vi "GUI MAIN.vi"() -> ()   [LabVIEW 2022 SP3]
uses:
  <vilib>/Instr/_visa.llb/VISA Configure Serial Port (Instr).vi
panel:
  out "Selected Freq":i32
  in  "Send":bool
  out "Send return count":u32
  in  "stop":bool
  in  "input cluster":T1
  out "read buffer":string
  out "return count":u32
  in  "VISA resource name":refnum<visa-resource-name>
  in  "FT DataSize":i32
  out "Fourier Transform":cluster{i32, dbl, i32[][]}(graph)
  out "Intensity Chart":i32[][](graph)
  out "Thermometer 5":i32(slide) scale=20.0..20000.0
  in  "Signal 5":bool
  out "Thermometer 4":i32(slide) scale=20.0..20000.0
  out "Thermometer 3":i32(slide) scale=20.0..20000.0
  out "Thermometer 2":i32(slide) scale=20.0..20000.0
  out "Thermometer 1":i32(slide) scale=20.0..20000.0
  in  "Signal 4":bool
  in  "Signal 3":bool
  in  "Signal 2":bool
  in  "Signal 1":bool
  out "Radar Graph":i32[][](graph)
  # "Signature Selection"
  # "Frequency (Hz)"
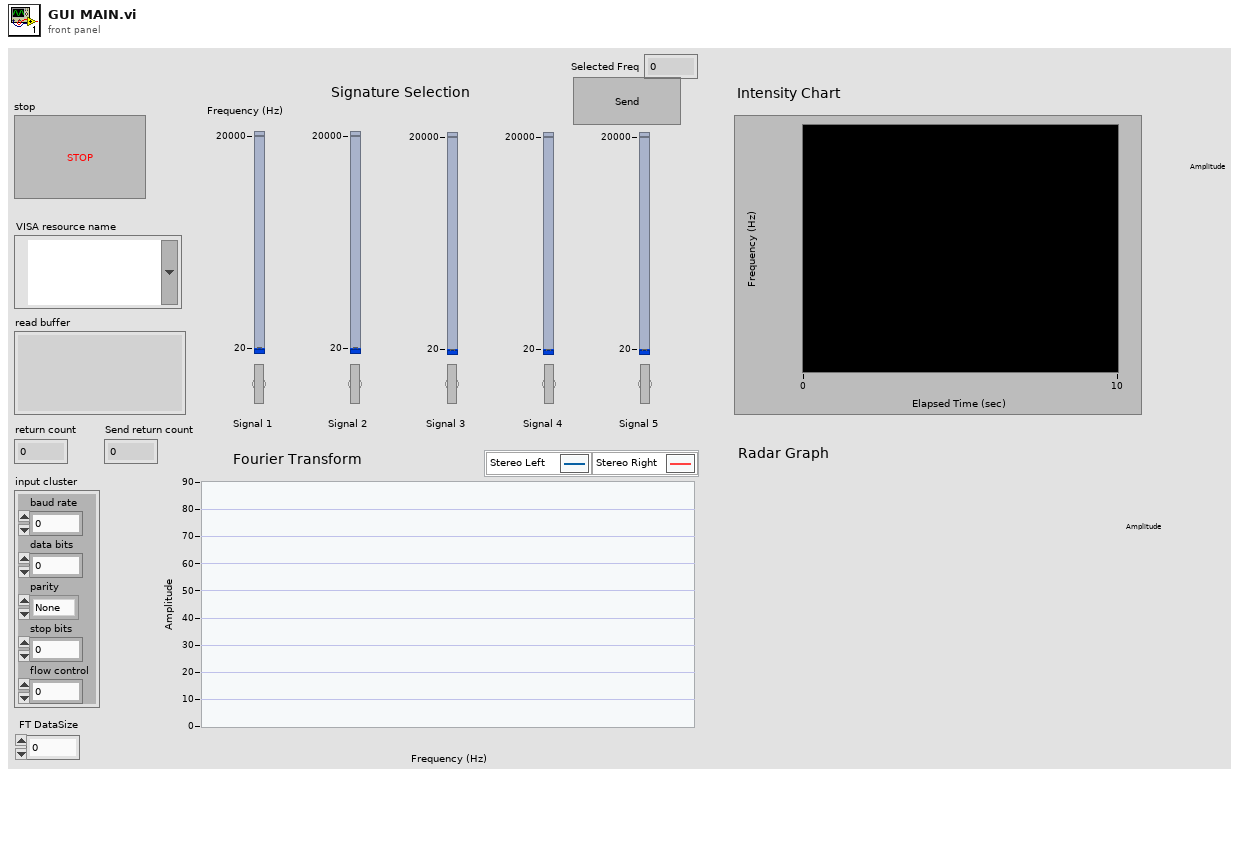
[diagram p1: front panel]
types:
  T1 = cluster{"baud rate":u32, "data bits":u16, "parity":enum16{"None", "Odd", "Even", "Mark", "Space"}, "stop bits":u16, "flow control":u16}
  T2 = cluster{"Width":u16, "Style":enum32{"Solid", "Dash", "Dot", "DashDot", "DashDotDot"}}
  T3 = typedef "LVRectTypeDef.ctl" = cluster{"left":i16, "top":i16, "right":i16, "bottom":i16}
  T4 = typedef "LVPoint32TypeDef.ctl" = cluster{"Horizontal":i32, "Vertical":i32}
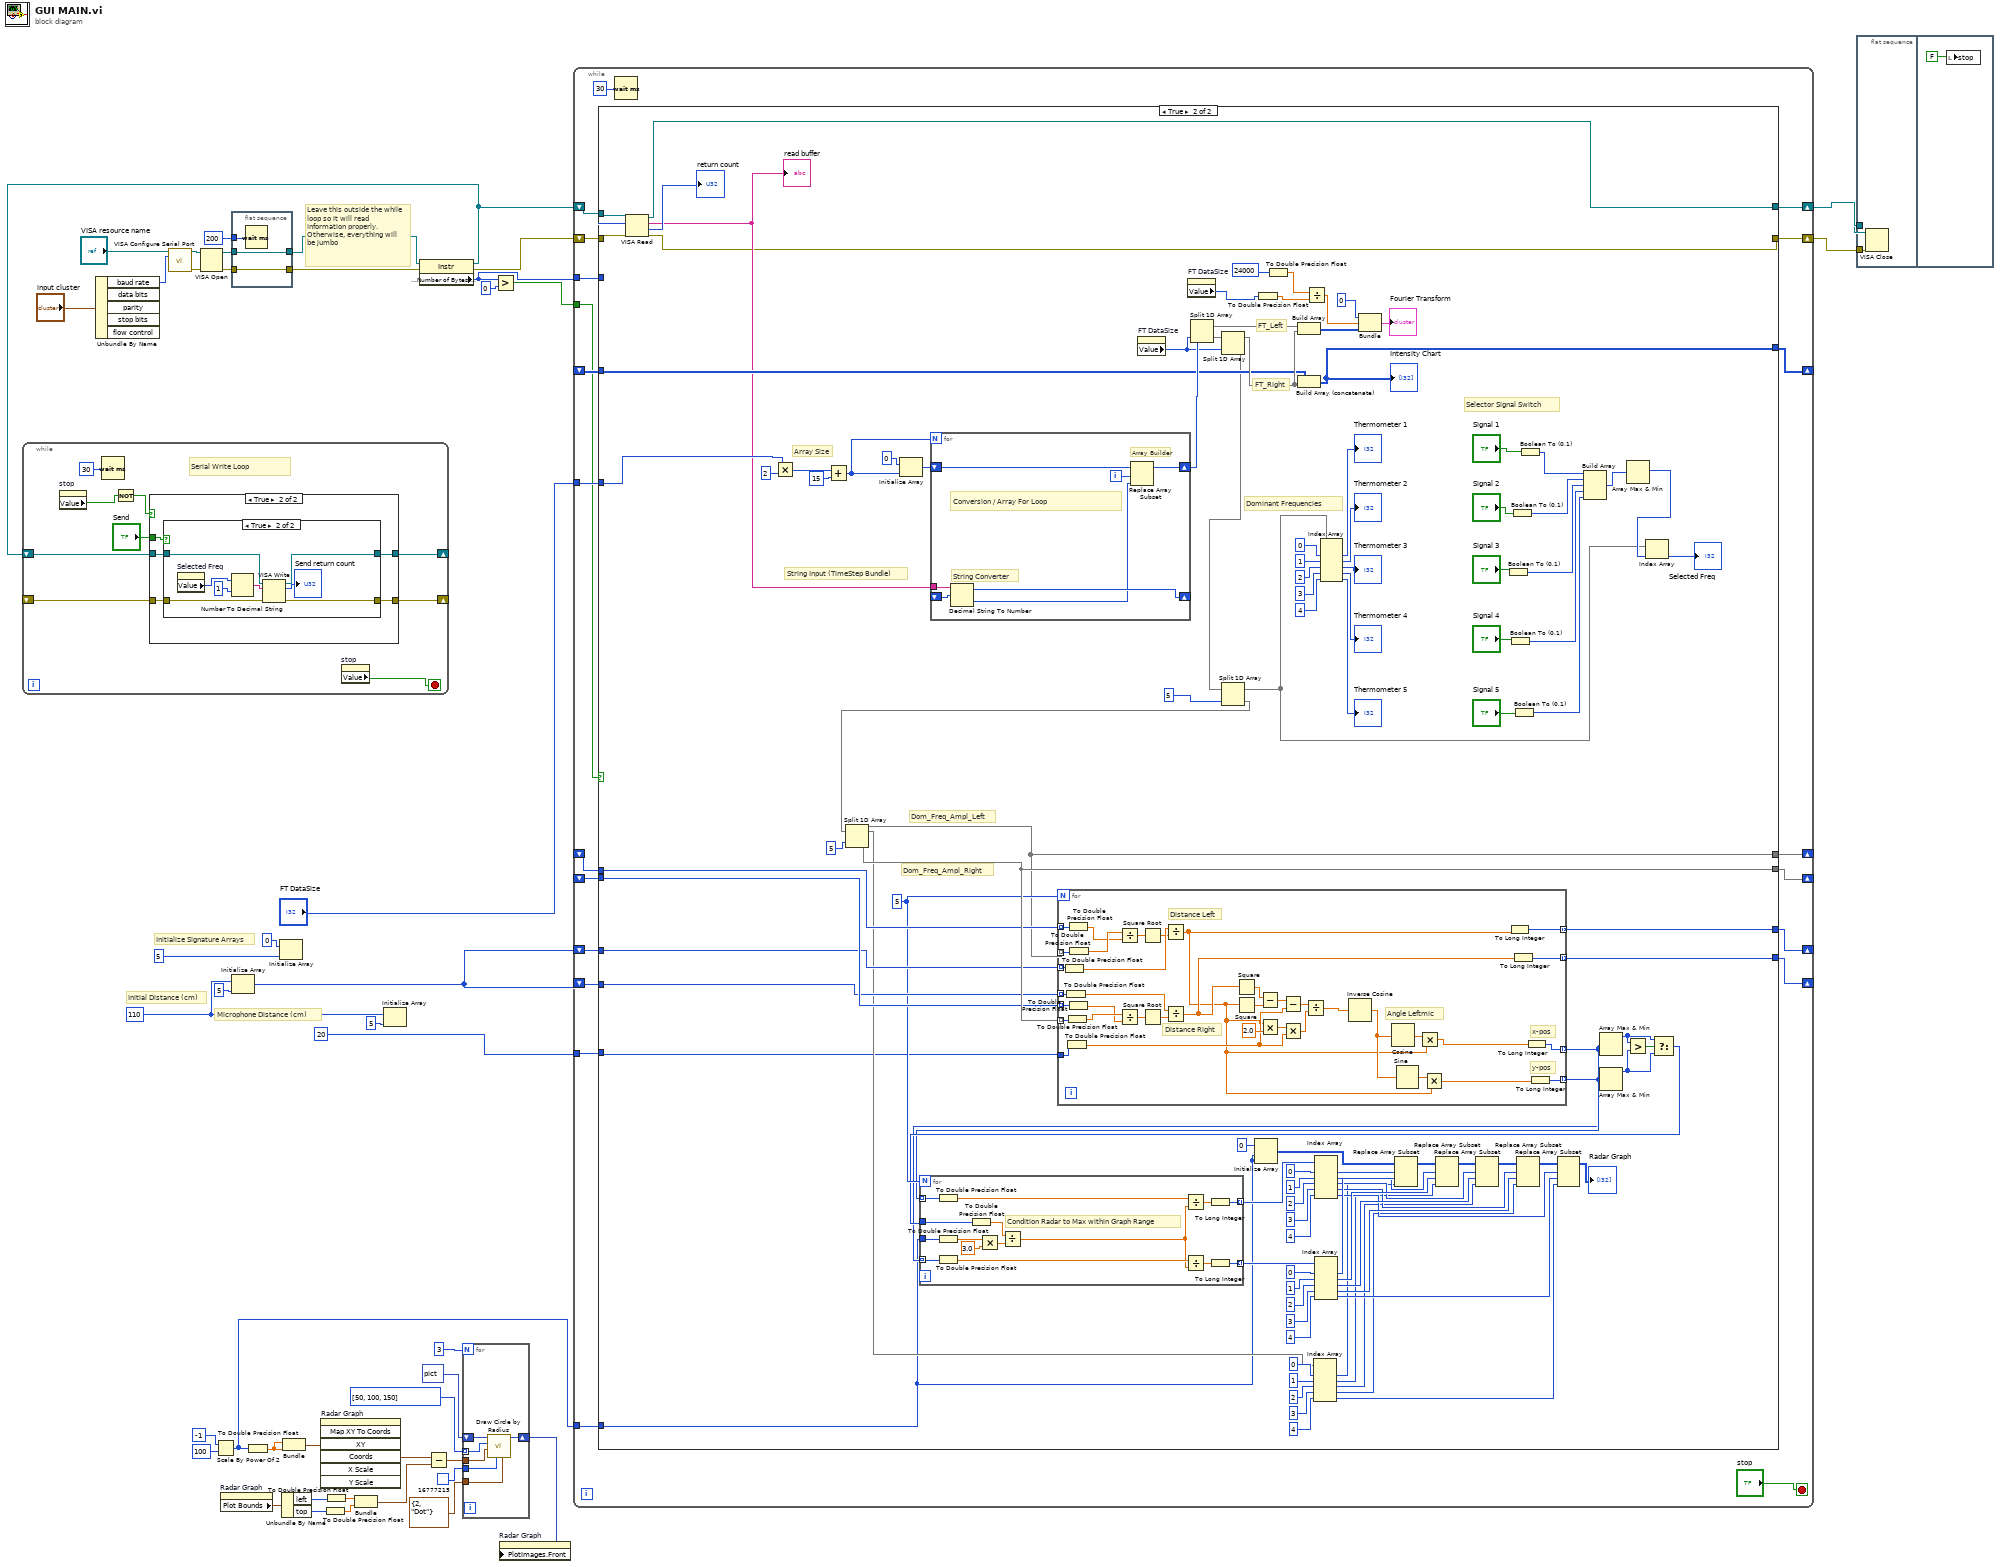
[diagram p0: block diagram]
diagram:
  w27 = 110
  # "Leave this outside the while loop so it will read information properly. Otherwise, everything will be jumbo"
  # "Initialize Signature Arrays"
  # "Microphone Distance (cm)"
  # "Initial Distance (cm)"
  n1 = Unbundle By Name("input cluster") -> ("baud rate"=w19:u32)  [unwired: 4 out]
  n2 = call-poly "VISA Configure Serial Port"("VISA resource name"="VISA resource name", "baud rate (9600)"=w19) -> ("VISA resource name out"=w17:refnum<visa-resource-name>, "error out"=w16:errorcluster)  [unwired: 12 in]
  n3 = VISA Open(error in (no error)=w16, VISA resource name=w17) -> (VISA resource name=w24:refnum<visa-resource-name>, error out=w23:errorcluster)  [unwired: 3 in]
  n4 = Scale By Power Of 2(n=-1, x=100 ("samples")) -> (x*2^n=w1:i32)
  n5 = property on="Radar Graph" class="IntGraph (strict)"() -> ("Plot Bounds"=w35:T3)  [unwired: 2 in, 2 out]
  n6 = flat-sequence {
    tunnel: w23 -> [w46]
    tunnel: [w46] -> w15
    tunnel: w24 -> [w45]
    tunnel: [w45] -> w20
    tunnel: u32 200 -> [w47]
    frame #0 {
      n7 = Wait (ms)(milliseconds to wait=w47) -> ()  [unwired: 1 out]
    }
  }
  n8 = Initialize Array(w27, 5) -> (w30:i32[])
  n9 = To Double Precision Float(number=w1) -> (double precision float=w8:dbl)
  n10 = Initialize Array(0, 5) -> ()  [unwired: 1 out]
  n11 = Unbundle By Name(w35) -> ("left"=w6:i16, "top"=w4:i16)
  n12 = Bundle(w8, w8) -> (w7:cluster{dbl, dbl})  [unwired: 1 in]
  n13 = invoke on="Radar Graph" class="IntGraph (strict)" method="Map XY To Coords"("XY"=w7) -> ("Coords"=w2:T4)  [unwired: 6 in, 6 out]
  n14 = To Double Precision Float(number=w4) -> (double precision float=w3:dbl)
  n15 = To Double Precision Float(number=w6) -> (double precision float=w5:dbl)
  n16 = Bundle(w5, w3) -> (w34:cluster{dbl, dbl})  [unwired: 1 in]
  n17 = Initialize Array(w27, 5) -> ()  [unwired: 1 out]
  n18 = property class="Instr"(reference=w20, error in=w15) -> (reference out=w9:refnum<visa-resource-name>, error out=w11:errorcluster, "Serial Settings:Number of Bytes at Serial Port"=w12:u32)
  n19 = while {
    shift-right: [w55] -> _
    shift-left: w9 -> [w56]
    shift-right: [w52] -> _
    shift-left: _ -> [w53]
    stop <- w48 stop-if-true
    # "Serial Write Loop"
    n20 = property on="stop" class="Bool (strict)"() -> ("Value"=w51:bool)  [unwired: 2 in, 2 out]
    n21 = Wait (ms)(milliseconds to wait=u32 30) -> ()  [unwired: 1 out]
    n22 = Not(x=w51) -> (.not. x?=w50:bool)
    n23 = case shown="True" w50 {
      tunnel: w56 -> [w58 w62]
      tunnel: [w58 w59] -> w55
      tunnel: w53 -> [w57 w61]
      tunnel: [w57 w60] -> w52
      tunnel: "Send" -> [_ w63]
      frame False {
      }
      frame True {
        n24 = case shown="True" w63 {
          tunnel: w62 -> [w65 w70]
          tunnel: w61 -> [w64 w69]
          tunnel: [w64 w67] -> w60
          tunnel: [w65 w68] -> w59
          frame False {
          }
          frame True {
            n25 = property on="Selected Freq" class="DigNum (strict)"() -> ("Value"=w66:i32)  [unwired: 2 in, 2 out]
            n26 = Number To Decimal String(number=w66, width (-)=i16 1) -> (decimal integer string=w72:string)
            n27 = VISA Write(VISA resource name=w70, write buffer=w72, error in (no error)=w69) -> (VISA resource name out=w68:refnum<visa-resource-name>, return count=→"Send return count":u32, error out=w67:errorcluster)
          }
        }
      }
    }
    n28 = property on="stop" class="Bool (strict)"() -> ("Value"=w48:bool)  [unwired: 2 in, 2 out]
  }
  n29 = Subtract(x=w2, y=w34) -> (x-y=w36:cluster{dbl, dbl})
  n30 = for {
    N: 3 -> [_]
    tunnel: w36 -> [w79]
    tunnel: u32 16777215 ("color(black)") -> [w78]
    tunnel: T2 {"Width"=2, "Style"=enum."Dot"} ("pen") -> [w77]
    tunnel: i16[] [50, 100, 150] -> [w76] mode=indexing
    shift-right: [w74] -> w38
    shift-left: picture data[5B] ("new picture") -> [w75]
    n31 = call <vilib>:"Draw Circle by Radius.vi"("pen"=w77, "color(black)"=w78, "pixel center"=w79, "radius"=w76, "picture"=w75) -> ("new picture"=w74:picture)  [unwired: 6 in]
  }
  n32 = Greater?(x=w12, y=u32 0) -> (0:w10:bool)
  n33 = property on="Radar Graph" class="IntGraph (strict)"("PlotImages.Front"=w38) -> ()  [unwired: 2 in, 2 out]
  n34 = while {
    shift-right: [w80] -> _
    shift-left: _ -> [w100]
    tunnel: "FT DataSize" -> [w99]
    tunnel: 20 -> [w83]
    shift-right: [w87] -> _
    shift-left: _ -> [w91]
    shift-right: [w86] -> _
    shift-left: _ -> [w92]
    shift-right: [w85] -> _
    shift-left: w30 -> [w90]
    shift-right: [w84] -> _
    shift-left: w30 -> [w89]
    shift-right: [w82] -> w14
    shift-left: w9 -> [w96]
    shift-right: [w81] -> w13
    shift-left: w11 -> [w95]
    tunnel: w12 -> [w94]
    tunnel: w10 -> [w93]
    tunnel: w1 -> [w88]
    stop <- "stop" stop-if-true
    n35 = case shown="True" w93 {
      tunnel: w100 -> [w105 w211]
      tunnel: [w105 w210] -> w80
      tunnel: w99 -> [_ w195]
      tunnel: [w103 w189] -> w86
      tunnel: w91 -> [w104 w188]
      tunnel: w92 -> [w103 w187]
      tunnel: w90 -> [w102 w186]
      tunnel: w89 -> [w101 w185]
      tunnel: [w101 w184] -> w84
      tunnel: [w102 w183] -> w85
      tunnel: w83 -> [_ w126]
      tunnel: [w104 w143] -> w87
      tunnel: w96 -> [w107 w131]
      tunnel: w95 -> [w106 w130]
      tunnel: w94 -> [_ w128]
      tunnel: w88 -> [_ w124]
      tunnel: [w107 w114] -> w82
      tunnel: [w106 w113] -> w81
      frame False {
      }
      frame True {
        w182 = 5
        # "String Input (TimeStep Bundle)"
        # "Selector Signal Switch"
        # "Dom_Freq_Ampl_Right"
        # "Dom_Freq_Ampl_Left"
        # "Dominant Frequencies"
        # "FT_Right"
        # "FT_Left"
        # "Array Size"
        n36 = VISA Read(VISA resource name=w131, byte count=w128, error in (no error)=w130) -> (VISA resource name out=w114:refnum<visa-resource-name>, read buffer=w125:string, return count=→"return count":u32, error out=w113:errorcluster)
        "read buffer" <- w125
        n37 = Multiply(x=w195, y=2) -> (x*y=w193:i32)
        n38 = Add(x=w193, y=15) -> (x+y=w191:i32)
        n39 = Initialize Array(0, w191) -> (w219:i32[])
        n40 = for {
          N: w191 -> [_]
          tunnel: w125 -> [w279]
          shift-right: [w278] -> _
          shift-left: _ -> [w277]
          shift-right: [w276] -> w218
          shift-left: w219 -> [w275]
          i -> [w273]
          # "String Converter"
          # "Array Builder"
          # "Conversion / Array For Loop"
          n41 = Decimal String To Number(string=w279, offset=w277) -> (offset past number=w278:i32, number=w274:i32)  [unwired: 1 in]
          n42 = Replace Array Subset(array=w275, new element=w274, index=w273) -> (w276:i32[])
        }
        n43 = property on="FT DataSize" class="DigNum (strict)"() -> ("Value"=w190:i32)  [unwired: 2 in, 2 out]
        n44 = property on="FT DataSize" class="DigNum (strict)"() -> ("Value"=w109:i32)  [unwired: 2 in, 2 out]
        n45 = Split 1D Array(array=w218, index=w190) -> (first subarray=w216:i32[], second subarray=w217:i32[])
        n46 = Split 1D Array(array=w217, index=w190) -> (first subarray=w212:i32[], second subarray=w199:i32[])
        n47 = Split 1D Array(array=w199, index=5) -> (first subarray=w116:i32[], second subarray=w196:i32[])
        n48 = Split 1D Array(array=w196, index=5) -> (first subarray=w143:i32[], second subarray=w189:i32[])
        n49 = for {
          N: w182 -> [_]
          tunnel: w143 -> [w270] mode=indexing
          tunnel: w189 -> [w269] mode=indexing
          tunnel: w188 -> [w272] mode=indexing
          tunnel: w187 -> [w271] mode=indexing
          tunnel: w186 -> [w262] mode=indexing
          tunnel: w185 -> [w261] mode=indexing
          tunnel: [w255] -> w184 mode=indexing
          tunnel: [w256] -> w183 mode=indexing
          tunnel: w126 -> [w254]
          tunnel: [w237] -> w177 mode=indexing
          tunnel: [w238] -> w176 mode=indexing
          # "y-pos"
          # "x-pos"
          # "Angle Leftmic"
          # "Distance Right"
          # "Distance Left"
          n50 = To Double Precision Float(number=w262) -> (double precision float=w260:dbl)
          n51 = To Double Precision Float(number=w261) -> (double precision float=w258:dbl)
          n52 = To Double Precision Float(number=w254) -> (double precision float=w247:dbl)
          n53 = To Double Precision Float(number=w269) -> (double precision float=w266:dbl)
          n54 = To Double Precision Float(number=w272) -> (double precision float=w267:dbl)
          n55 = To Double Precision Float(number=w271) -> (double precision float=w265:dbl)
          n56 = To Double Precision Float(number=w270) -> (double precision float=w268:dbl)
          n57 = Divide(x=w268, y=w267) -> (x/y=w263:dbl)
          n58 = Divide(x=w266, y=w265) -> (x/y=w264:dbl)
          n59 = Square Root(x=w263) -> (sqrt(x)=w259:dbl)
          n60 = Square Root(x=w264) -> (sqrt(x)=w257:dbl)
          n61 = Divide(x=w260, y=w259) -> (x/y=w240:dbl)
          n62 = Divide(x=w258, y=w257) -> (x/y=w253:dbl)
          n63 = Square(x=w253) -> (x^2=w252:dbl)
          n64 = Square(x=w240) -> (x^2=w251:dbl)
          n65 = Subtract(x=w252, y=w251) -> (x-y=w250:dbl)
          n66 = Multiply(x=w240, y=2.0) -> (x*y=w248:dbl)
          n67 = Subtract(x=w250, y=w247) -> (x-y=w246:dbl)
          n68 = Multiply(x=w248, y=w247) -> (x*y=w245:dbl)
          n69 = Divide(x=w246, y=w245) -> (x/y=w244:dbl)
          n70 = Inverse Cosine(1:w244) -> (0:w243:dbl)
          n71 = Cosine(x=w243) -> (cos(x)=w242:dbl)
          n72 = Sine(x=w243) -> (sin(x)=w241:dbl)
          n73 = Multiply(x=w242, y=w240) -> (x*y=w236:dbl)
          n74 = Multiply(x=w241, y=w240) -> (x*y=w239:dbl)
          n75 = To Long Integer(number=w240) -> (32bit integer=w256:i32)
          n76 = To Long Integer(number=w253) -> (32bit integer=w255:i32)
          n77 = To Long Integer(number=w236) -> (32bit integer=w237:i32)
          n78 = To Long Integer(number=w239) -> (32bit integer=w238:i32)
        }
        n79 = Initialize Array(0, w124, w124) -> (w163:i32[][])
        n80 = To Double Precision Float(number=w109) -> (double precision float=w108:dbl)
        n81 = To Double Precision Float(number=24000) -> (double precision float=w110:dbl)
        n82 = Build Array(w216, w212) -> (w215:i32[][])
        n83 = Build Array (concatenate)(w211, w212) -> (w210:i32[][])
        "Intensity Chart" <- w210
        n84 = Divide(x=w110, y=w108) -> (x/y=w112:dbl)
        n85 = Index Array(array=w143, index #1=0, index #2=1, index #3=2, index #4=3, index #5=4) -> (element #1=w142:i32, element #2=w141:i32, element #3=w140:i32, element #4=w139:i32, element #5=w138:i32)
        n86 = Index Array(array=w116, index #1=0, index #2=1, index #3=2, index #4=3, index #5=4) -> (element #1=→"Thermometer 1":i32, element #2=→"Thermometer 2":i32, element #3=→"Thermometer 3":i32, element #4=→"Thermometer 4":i32, element #5=→"Thermometer 5":i32)
        n87 = Bundle(0, w112, w215) -> (→"Fourier Transform":cluster{i32, dbl, i32[][]})  [unwired: 1 in]
        n88 = Boolean To (0,1)(Boolean="Signal 3") -> (0, 1=w121:i16)
        n89 = Boolean To (0,1)(Boolean="Signal 4") -> (0, 1=w120:i16)
        n90 = Boolean To (0,1)(Boolean="Signal 2") -> (0, 1=w122:i16)
        n91 = Boolean To (0,1)(Boolean="Signal 5") -> (0, 1=w119:i16)
        n92 = Boolean To (0,1)(Boolean="Signal 1") -> (0, 1=w123:i16)
        n93 = Build Array(w123, w122, w121, w120, w119) -> (w118:i16[])
        n94 = Array Max & Min(array=w177) -> (max value=w180:i32)  [unwired: 3 out]
        n95 = Array Max & Min(array=w176) -> (max value=w179:i32)  [unwired: 3 out]
        n96 = Array Max & Min(array=w118) -> (max index (indices)=w117:i32)  [unwired: 3 out]
        n97 = Greater?(x=w180, y=w179) -> (0:w181:bool)
        n98 = Index Array(array=w116, index=w117) -> (element=→"Selected Freq":i32)
        n99 = Select(t=w180, s=w181, f=w179) -> (s? t:f=w178:i32)
        n100 = for {
          N: w182 -> [_]
          tunnel: w178 -> [w235]
          tunnel: w177 -> [w231] mode=indexing
          tunnel: w176 -> [w232] mode=indexing
          tunnel: w124 -> [w234]
          tunnel: [w225] -> w165 mode=indexing
          tunnel: [w224] -> w127 mode=indexing
          # "Condition Radar to Max within Graph Range"
          n101 = To Double Precision Float(number=w231) -> (double precision float=w230:dbl)
          n102 = To Double Precision Float(number=w234) -> (double precision float=w223:dbl)
          n103 = To Double Precision Float(number=w232) -> (double precision float=w229:dbl)
          n104 = To Double Precision Float(number=w235) -> (double precision float=w233:dbl)
          n105 = Multiply(x=w223, y=3.0) -> (x*y=w221:dbl)
          n106 = Divide(x=w233, y=w221) -> (x/y=w228:dbl)
          n107 = Divide(x=w230, y=w228) -> (x/y=w227:dbl)
          n108 = Divide(x=w229, y=w228) -> (x/y=w226:dbl)
          n109 = To Long Integer(number=w227) -> (32bit integer=w225:i32)
          n110 = To Long Integer(number=w226) -> (32bit integer=w224:i32)
        }
        n111 = Index Array(array=w165, index #1=0, index #2=1, index #3=2, index #4=3, index #5=4) -> (element #1=w162:i32, element #2=w160:i32, element #3=w158:i32, element #4=w156:i32, element #5=w154:i32)
        n112 = Index Array(array=w127, index #1=0, index #2=1, index #3=2, index #4=3, index #5=4) -> (element #1=w161:i32, element #2=w159:i32, element #3=w157:i32, element #4=w155:i32, element #5=w153:i32)
        n113 = Replace Array Subset(array=w163, new element=w142, index (row)=w162, index (col)=w161) -> (w152:i32[][])
        n114 = Replace Array Subset(array=w152, new element=w141, index (row)=w160, index (col)=w159) -> (w151:i32[][])
        n115 = Replace Array Subset(array=w151, new element=w140, index (row)=w158, index (col)=w157) -> (w150:i32[][])
        n116 = Replace Array Subset(array=w150, new element=w139, index (row)=w156, index (col)=w155) -> (w149:i32[][])
        n117 = Replace Array Subset(array=w149, new element=w138, index (row)=w154, index (col)=w153) -> (→"Radar Graph":i32[][])
      }
    }
    n118 = Wait (ms)(milliseconds to wait=u32 30) -> ()  [unwired: 1 out]
  }
  n119 = flat-sequence {
    tunnel: w13 -> [w281]
    tunnel: w14 -> [w280]
    frame #0 {
      n120 = VISA Close(VISA resource name=w280, error in (no error)=w281) -> ()  [unwired: 1 out]
    }
    frame #1 {
      n121 = local write "stop"(FALSE) -> ()
    }
  }
